vi "Get Bond Pad Local Coordinates.vi"(8 "error in":errorcluster, 9 "ROC":i32, 10 "Part Type":T1, 11 "Config Manager":refnum<class "Config Manager Class.lvclass">) -> (0 "error out":errorcluster, 2 "Pad Local Coordinates":refnum<class "Vec3d Class.lvclass">)   [LabVIEW 2011]
uses:
  Vec3d Class/Vec3d Class.lvclass
  Config Manager Class/Config Manager Class.lvclass
  Config Manager Class/Type Definitions/Part Type.ctl
  Config Manager Class/Read Geometry Definition 3D.vi
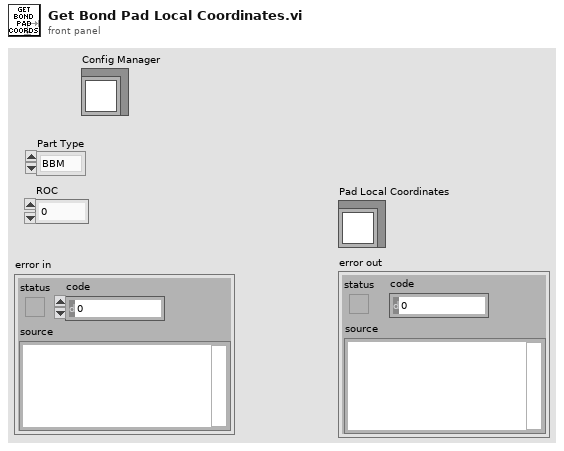
[diagram p1: front panel]
types:
  T1 = typedef "Part Type.ctl" = enum16{"BBM", "HDI", "GLUERESERVOIR", "STAMP", "WEIGHT"}
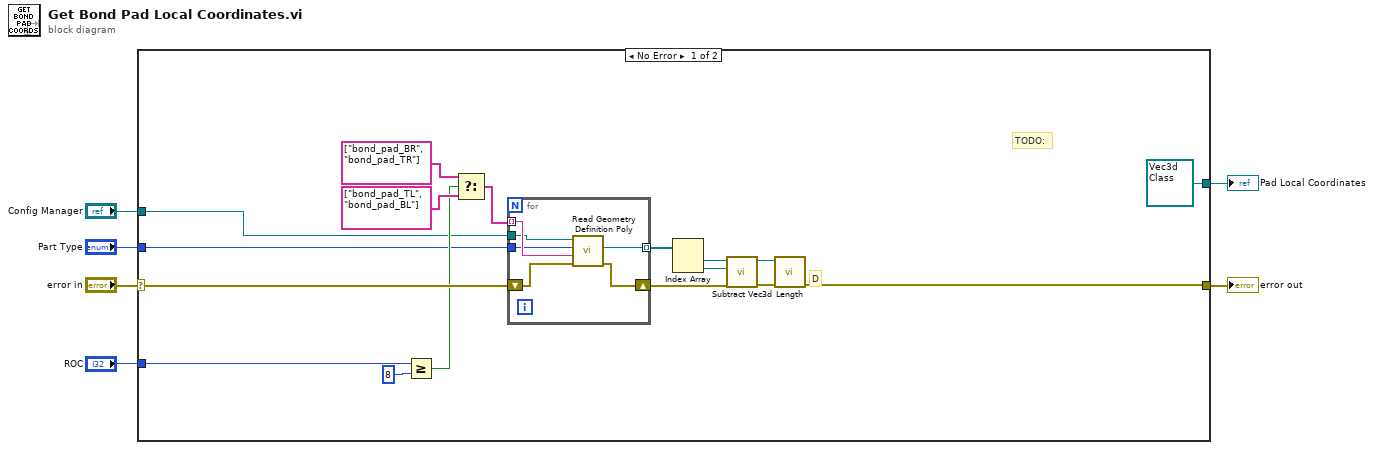
[diagram p0: block diagram]
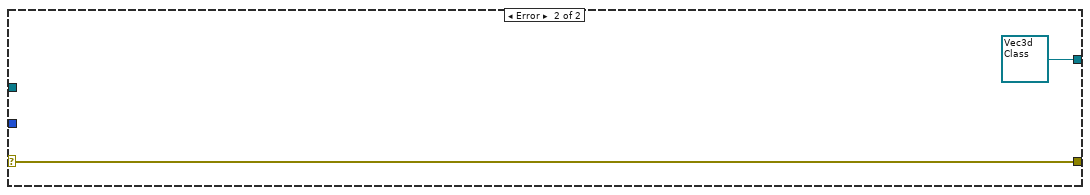
[diagram p2: hidden frame]
diagram:
  n1 = case shown="No Error" "error in" {
    selector: "error in" -> [w23 w31]
    tunnel: "ROC" -> [w17 _]
    tunnel: [refnum<class "Vec3d Class.lvclass"> refnum ("Vec3d Class out") refnum<class "Vec3d Class.lvclass"> refnum ("Vec3d Class out")] -> w5
    tunnel: [w7 w31] -> w4
    tunnel: "Part Type" -> [w15 _]
    tunnel: "Config Manager" -> [w14 _]
    frame No Error {
      # "TODO:"
      # "D"
      n2 = Greater Or Equal?(x=w17, y=8 ("x")) -> (x >= y?=w19:bool)
      n3 = Select(t=string[] ["bond_pad_BR", "bond_pad_TR"], s=w19, f=string[] ["bond_pad_TL", "bond_pad_BL"]) -> (s? t:f=w22:string[])
      n4 = for {
        shift-right: [w25] -> w10
        shift-left: w23 -> [w26]
        tunnel: w22 -> [w29] mode=indexing
        tunnel: w15 -> [w27]
        tunnel: w14 -> [w28]
        tunnel: [w24] -> w13 mode=indexing
        n5 = call-poly "Read Geometry Definition Poly.vi"("error in"=w26, "Feature"=w29, "Part Type"=w27, "Config Manager in"=w28) -> ("error out"=w25:errorcluster, "Feature Coordinates"=w24:refnum<class "Vec3d Class.lvclass">)  [unwired: 5 in, 1 out]
      }
      n6 = Index Array(array=w13) -> (element #1=w12:refnum<class "Vec3d Class.lvclass">, element #2=w11:refnum<class "Vec3d Class.lvclass">)  [unwired: 2 in]
      n7 = call "Subtract Vec3d.vi"("error in (no error)"=w10, "Vec3d in 2"=w11, "Vec3d in 1"=w12) -> ("error out"=w9:errorcluster, "Vec3d Class out"=w16:refnum<class "Vec3d Class.lvclass">)  [unwired: 7 in]
      n8 = call-dynamic "Length.vi"("error in"=w9, "Vec3d in"=w16) -> ("error out"=w7:errorcluster)  [unwired: 7 in, 2 out]
    }
    frame Error {
    }
  }
  "Pad Local Coordinates" <- w5
  "error out" <- w4
